vi "BoundsToOffsetedBounds.vi"(9 "Offset":T1, 10 "Bounds":T2) -> (2 "Bounds + Offset":T2)   [LabVIEW 2023]
doc: "This VI gets bounds data and moves it's position by Offset."
uses:
  <vilib>/Utility/miscctls.llb/LVRectTypeDef.ctl
  <vilib>/Utility/miscctls.llb/LVPositionTypeDef.ctl
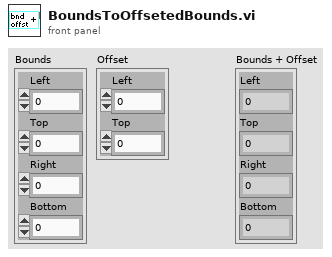
[diagram p1: front panel]
types:
  T1 = typedef "LVPositionTypeDef.ctl" = cluster{"Left":i32, "Top":i32}
  T2 = typedef "LVRectTypeDef.ctl" = cluster{"Left":i16, "Top":i16, "Right":i16, "Bottom":i16}
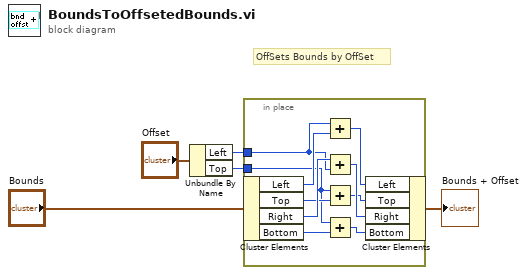
[diagram p0: block diagram]
diagram:
  # "OffSets Bounds by OffSet"
  n1 = Unbundle By Name("Offset") -> ("Left"=w3:i32, "Top"=w2:i32)
  n2 = in-place "In Place Element Structure" {
    in-place-border: w3 -> [w7]
    in-place-border: w2 -> [w6]
    n3 = in-place-cluster #1("Bounds") -> ("Left"=w15:i16, "Top"=w9:i16, "Right"=w13:i16, "Bottom"=w8:i16)
    n4 = Add(x=w7, y=w15) -> (x+y=w14:i32)
    n5 = Add(x=w13, y=w7) -> (x+y=w12:i32)
    n6 = Add(x=w6, y=w9) -> (x+y=w11:i32)
    n7 = Add(x=w6, y=w8) -> (x+y=w10:i32)
    n8 = in-place-cluster #1("Left"=w14, "Top"=w11, "Right"=w12, "Bottom"=w10) -> (→"Bounds + Offset":T2)
  }
